vi "Close Motor Communication_Scalar.vi"(8 "error in (no error)":errorcluster, 11 "motor communication in":refnum<class "NI_Robotics_Motor Communication.lvclass">) -> (0 "error out":errorcluster)   [LabVIEW 2017, in "NI_Robotics_Motor Communication.lvclass"]
doc: "Terminates a communication session between a motor and the wheel the motor controls. Wire data to the <B>motor communication in</B> input to determine the polymorphic instance to use or manually select the instance."
uses:
  <vilib>/robotics/Actuation/Motor Communication/NI_Robotics_Motor Communication.lvclass
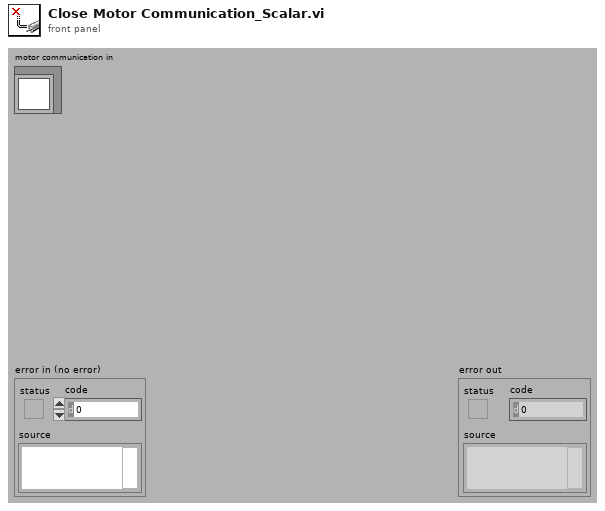
[diagram p1: front panel]
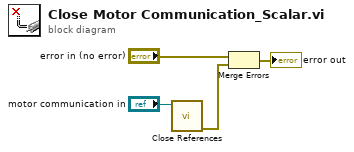
[diagram p0: block diagram]
diagram:
  n1 = call-dynamic "Close References.vi"("motor communication in"="motor communication in") -> ("error out"=w1:errorcluster)  [unwired: 10 in]
  n2 = Merge Errors("error in (no error)", w1) -> (→"error out":errorcluster)
